vi "OutBitStayInState.vi"(10 "OutBitsStateBefore":T1) -> (2 "OutBitsStateNext":T1)   [LabVIEW 2014]
uses:
  OutbitsStateControl.ctl
  <vilib>/rvi/Emulation/niFpgaGetClockAttributes.vi
  <vilib>/rvi/Emulation/niFpgaSctlEmulationGetInTimedLoop.vi
  <vilib>/rvi/Emulation/niFpgaEmulationReportErrorSimple.vi
  OutbitsGlobalVars.vi
  <vilib>/rvi/Emulation/niFpgaCriticalErrorInLSC.vi
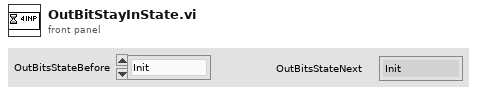
[diagram p1: front panel]
types:
  T1 = typedef "OutbitsStateControl.ctl" = enum16{"Init", "Idle", "loading", "listening", "clearing", "error"}
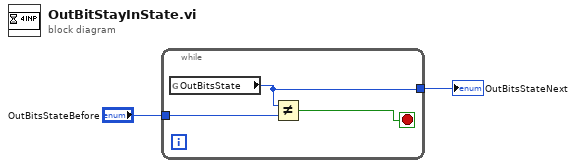
[diagram p0: block diagram]
diagram:
  n1 = while {
    tunnel: "OutBitsStateBefore" -> [w5]
    tunnel: [w3] -> w2
    stop <- w4 stop-if-true
    n2 = global read "OutbitsGlobalVars.vi" "OutBitsState"() -> (w3:T1)
    n3 = Not Equal?(x=w3, y=w5) -> (x != y?=w4:bool)
  }
  "OutBitsStateNext" <- w2
